vi "HatchLatch_slnd.vi"(11 "Toggle?":bool) -> ()   [LabVIEW 2018]
uses:
  <vilib>/Rock Robotics/WPI/Solenoid/Deprecated/WPI_SolenoidSetBool.vi
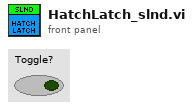
[diagram p1: front panel]
types:
  T1 = typedef "WPI_SolenoidDevRef.ctl" = cluster{"DevStatus":errorcluster, "Pneumatics Control Module":u8, "Forward Solenoid Channel":T2, "Reverse Solenoid Channel":T2}
  T2 = typedef "WPI_SolenoidChannel.ctl" = enum8{"Solenoid 0", "Solenoid 1", "Solenoid 2", "Solenoid 3", "Solenoid 4", "Solenoid 5", "Solenoid 6", "Solenoid 7", "Invalid"}
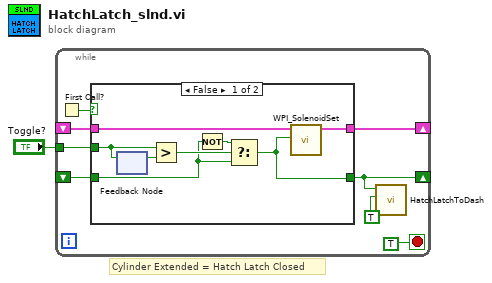
[diagram p0: block diagram]
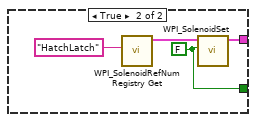
[diagram p2: hidden frame]
diagram:
  # "Cylinder Extended = Hatch Latch Closed"
  n1 = while {
    tunnel: "Toggle?" -> [w9]
    shift-right: [w7] -> _
    shift-left: _ -> [w6]
    shift-right: [w3] -> _
    shift-left: _ -> [w4]
    stop <- TRUE stop-if-true
    n2 = First Call?() -> (First Call?: T/F=w5:bool)
    n3 = case shown="False" w5 {
      tunnel: w9 -> [w12 _]
      tunnel: [w17 w20] -> w7
      tunnel: w6 -> [w16 _]
      tunnel: [w11 w18] -> w3
      tunnel: w4 -> [w10 _]
      frame False {
        n4 = feedback #1() -> (w15:bool)  [unwired: 1 in]
        n5 = feedback-in #1(w12) -> ()
        n6 = Greater?(x=w12, y=w15) -> (0:w14:bool)
        n7 = Not(x=w10) -> (.not. x?=w13:bool)
        n8 = Select(t=w13, s=w14, f=w10) -> (s? t:f=w11:bool)
        n9 = call-poly <vilib>:"WPI_SolenoidSet.vi"("Value"=w11, "SolenoidDevRef"=w16) -> ("SolenoidDevRef"=w17:T1)  [unwired: 8 in, 1 out]
      }
      frame True {
        w18 = FALSE
        n10 = call <vilib>:"WPI_SolenoidRefNum Registry Get.vi"("refnum name"="HatchLatch") -> ("SolenoidDevRef"=w19:T1)  [unwired: 9 in, 1 out]
        n11 = call-poly <vilib>:"WPI_SolenoidSet.vi"("Value"=w18, "SolenoidDevRef"=w19) -> ("SolenoidDevRef"=w20:T1)  [unwired: 8 in, 1 out]
      }
    }
    n12 = call "HatchLatchToDash.vi"("Update?"=TRUE, "HatchLatchIn"=w3) -> ()  [unwired: 9 in, 1 out]
  }
